vi "MeasureGrowthTrends.vi"(8 "Fixed":T1={"FixedDays"=FALSE, "DaysBack"=7, "FixTrendDays"=FALSE, "DaysBackTrend"=0}, 11 "Data":cluster{"Cases":i32[], "Days":timestamp[]}={"Cases"=[0, 0, 0, 0, 2, 2, 2, 2, 2, 3, 3, 3, 6, 6, 6, 6, 6, 6, 6, 6, 7, 7, 8, 8, 8, 8, 8, 8, 8, 8, 10, 10, 10, 10, 10, 10, 11, 11, 12, 12, 21, 25, 35, 51, 59, 102, 116, 167, 179, 247, 250, 305, 372, 480, 588, 741, 892, 1065, 1289, 1524, 1826, 2253, 2641, 3176, 4035, 4863, 5671, 6352, 7412, 8570, 9939, 11170, 12563, 13886], "Days"=[timestamp(3662524800 s since 1904-01-01), timestamp(3662611200 s since 1904-01-01), timestamp(3662697600 s since 1904-01-01), timestamp(3662784000 s since 1904-01-01), timestamp(3662870400 s since 1904-01-01), timestamp(3662956800 s since 1904-01-01), timestamp(3663043200 s since 1904-01-01), timestamp(3663129600 s since 1904-01-01), timestamp(3663216000 s since 1904-01-01), timestamp(3663302400 s since 1904-01-01), timestamp(3663388800 s since 1904-01-01), timestamp(3663475200 s since 1904-01-01), timestamp(3663561600 s since 1904-01-01), timestamp(3663648000 s since 1904-01-01), timestamp(3663734400 s since 1904-01-01), timestamp(3663820800 s since 1904-01-01), timestamp(3663907200 s since 1904-01-01), timestamp(3663993600 s since 1904-01-01), timestamp(3664080000 s since 1904-01-01), timestamp(3664166400 s since 1904-01-01), timestamp(3664252800 s since 1904-01-01), timestamp(3664339200 s since 1904-01-01), timestamp(3664425600 s since 1904-01-01), timestamp(3664512000 s since 1904-01-01), timestamp(3664598400 s since 1904-01-01), timestamp(3664684800 s since 1904-01-01), timestamp(3664771200 s since 1904-01-01), timestamp(3664857600 s since 1904-01-01), timestamp(3664944000 s since 1904-01-01), timestamp(3665030400 s since 1904-01-01), timestamp(3665116800 s since 1904-01-01), timestamp(3665203200 s since 1904-01-01), timestamp(3665289600 s since 1904-01-01), timestamp(3665376000 s since 1904-01-01), timestamp(3665462400 s since 1904-01-01), timestamp(3665548800 s since 1904-01-01), timestamp(3665635200 s since 1904-01-01), timestamp(3665721600 s since 1904-01-01), timestamp(3665808000 s since 1904-01-01), timestamp(3665894400 s since 1904-01-01), timestamp(3665980800 s since 1904-01-01), timestamp(3666067200 s since 1904-01-01), timestamp(3666153600 s since 1904-01-01), timestamp(3666240000 s since 1904-01-01), timestamp(3666326400 s since 1904-01-01), timestamp(3666412800 s since 1904-01-01), timestamp(3666499200 s since 1904-01-01), timestamp(3666585600 s since 1904-01-01), timestamp(3666672000 s since 1904-01-01), timestamp(3666758400 s since 1904-01-01), timestamp(3666844800 s since 1904-01-01), timestamp(3666931200 s since 1904-01-01), timestamp(3667017600 s since 1904-01-01), timestamp(3667104000 s since 1904-01-01), timestamp(3667190400 s since 1904-01-01), timestamp(3667276800 s since 1904-01-01), timestamp(3667363200 s since 1904-01-01), timestamp(3667449600 s since 1904-01-01), timestamp(3667536000 s since 1904-01-01), timestamp(3667622400 s since 1904-01-01), timestamp(3667708800 s since 1904-01-01), timestamp(3667795200 s since 1904-01-01), timestamp(3667881600 s since 1904-01-01), timestamp(3667968000 s since 1904-01-01), timestamp(3668054400 s since 1904-01-01), timestamp(3668140800 s since 1904-01-01), timestamp(3668227200 s since 1904-01-01), timestamp(3668313600 s since 1904-01-01), timestamp(3668400000 s since 1904-01-01), timestamp(3668486400 s since 1904-01-01), timestamp(3668572800 s since 1904-01-01), timestamp(3668659200 s since 1904-01-01), timestamp(3668745600 s since 1904-01-01), timestamp(3668832000 s since 1904-01-01)]}) -> (0 "Trend":cluster{"Days":timestamp[], dbl[]}[](graph), 1 "Growth":cluster{"Days":timestamp[], dbl[]}[](graph), 3 "Measure":T2={"Trend"=0.0, "TrendBest"=0.0, "TrendWorst"=0.0, "BestDays"=0.0, "WorstDays"=0.0, "Days"=0.0, "Growth"=16.31168636482856, "PlusMinus"=2.4408305776857144, "Cases"=0})   [LabVIEW 2017]
panel:
  out "GrowthError":dbl
  out "Growth":dbl
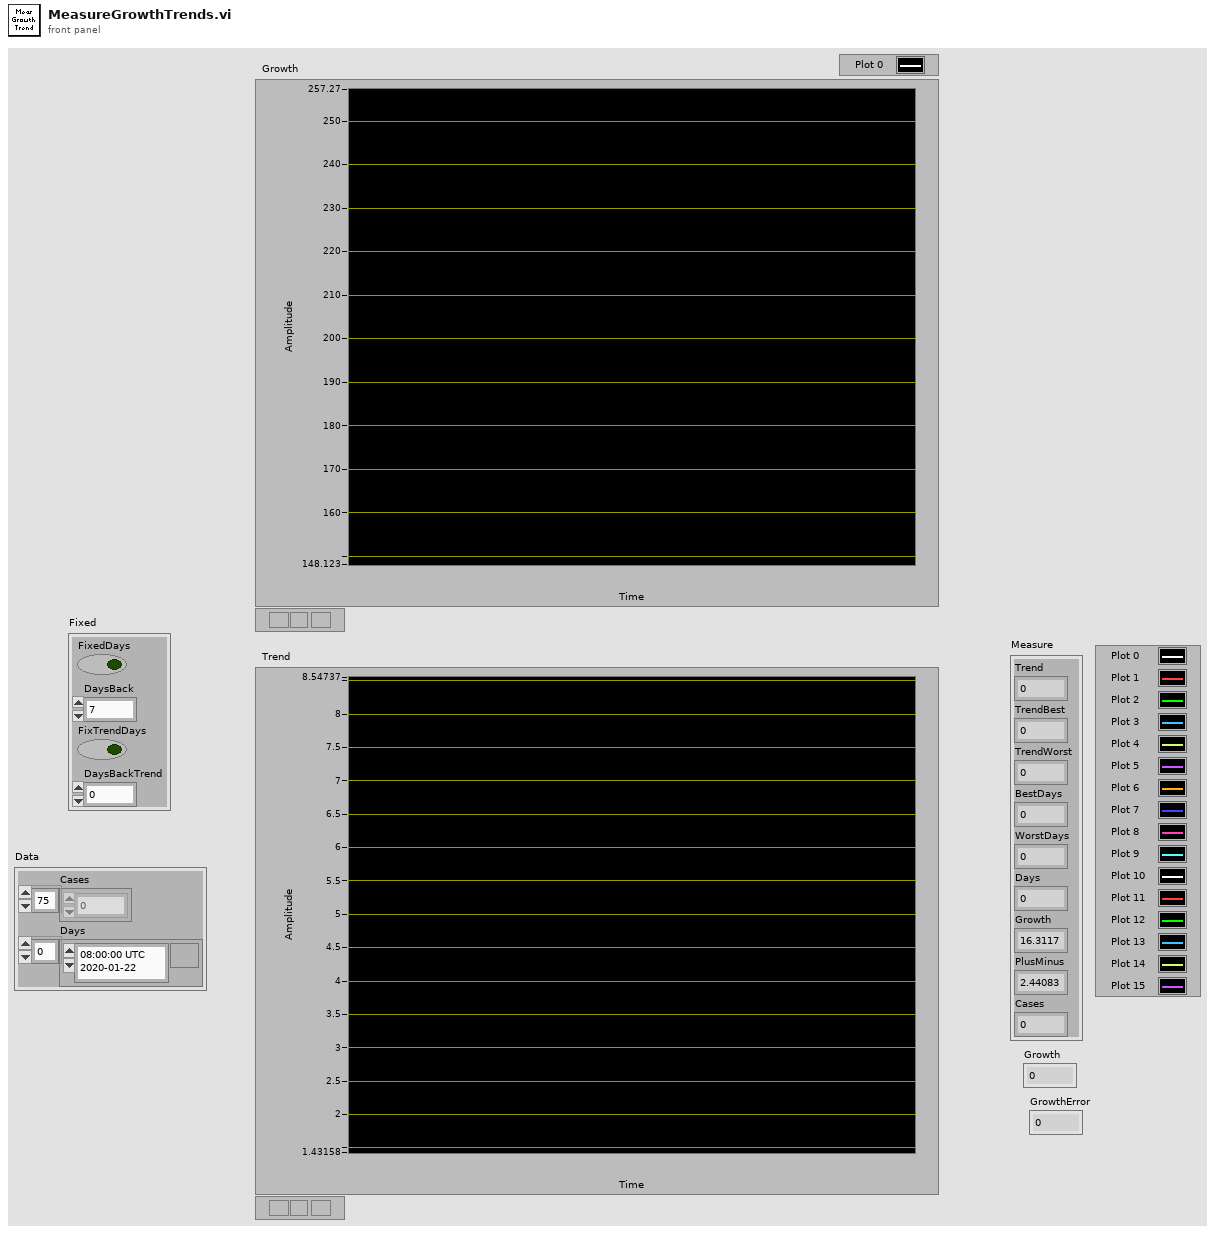
[diagram p1: front panel]
types:
  T1 = cluster{"FixedDays":bool, "DaysBack":i32, "FixTrendDays":bool, "DaysBackTrend":i32}
  T2 = cluster{"Trend":dbl, "TrendBest":dbl, "TrendWorst":dbl, "BestDays":dbl, "WorstDays":dbl, "Days":dbl, "Growth":dbl, "PlusMinus":dbl, "Cases":i32}
  T3 = cluster{"Days":timestamp[], "ConfirmedCases":dbl[]}[]
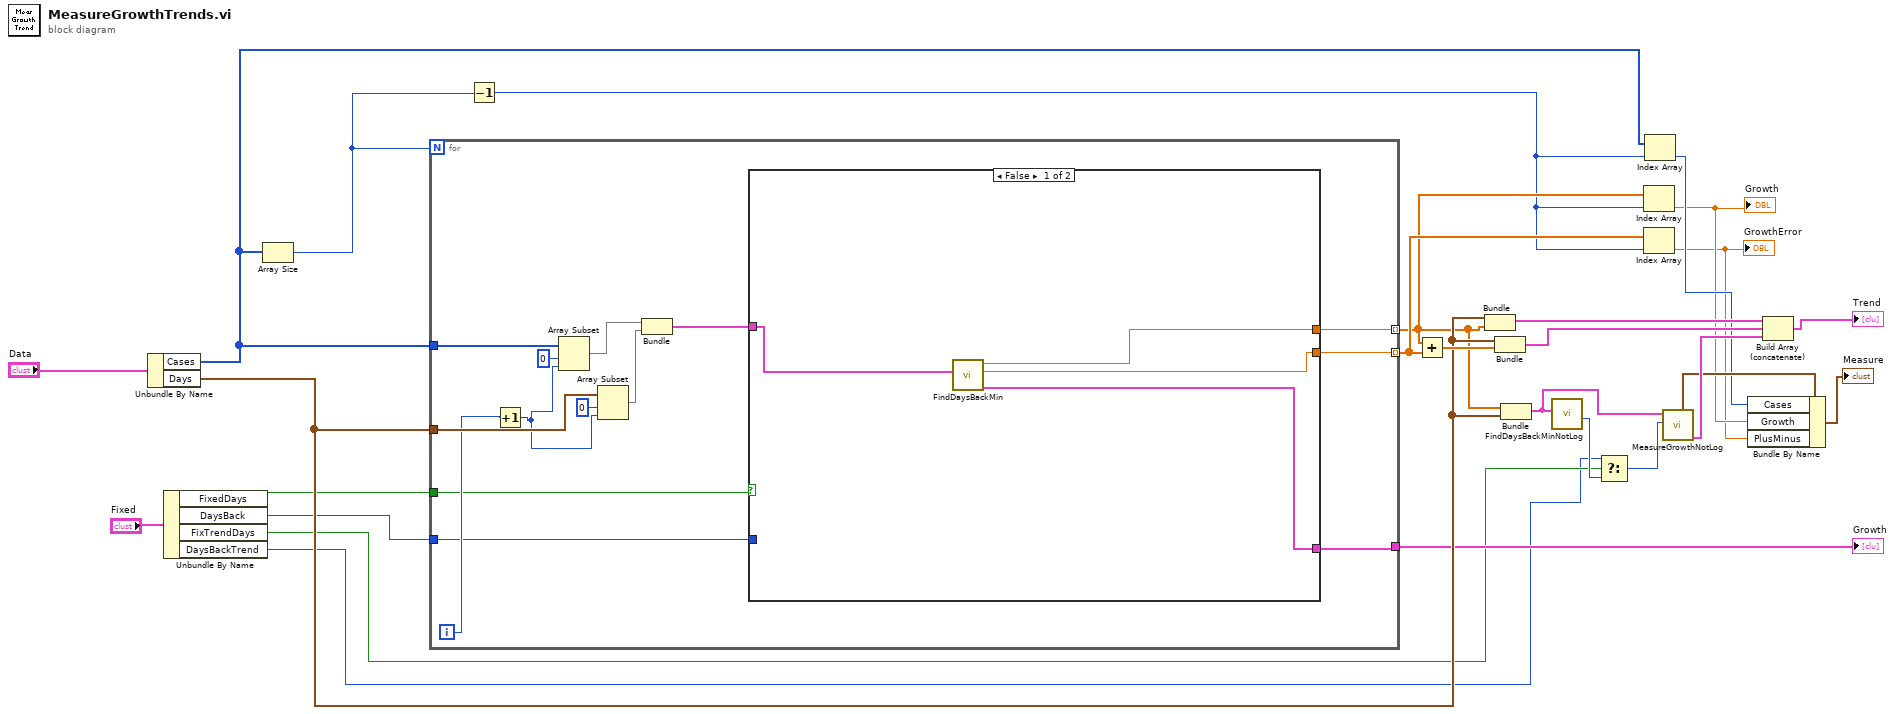
[diagram p0: block diagram]
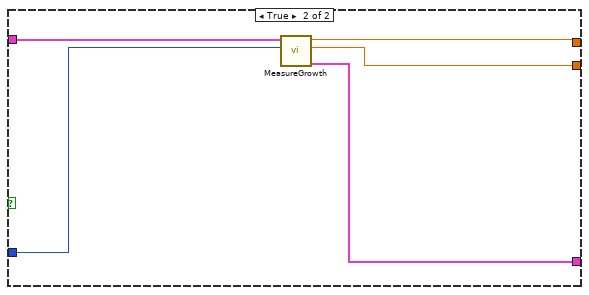
[diagram p2: hidden frame]
diagram:
  n1 = Unbundle By Name("Data") -> ("Cases"=w11:i32[], "Days"=w22:timestamp[])
  n2 = Unbundle By Name("Fixed") -> ("FixedDays"=w4:bool, "DaysBack"=w3:i32, "FixTrendDays"=w2:bool, "DaysBackTrend"=w1:i32)
  n3 = Array Size(array=w11) -> (size(s)=w20:i32)
  n4 = for {
    N: w20 -> [_]
    tunnel: w11 -> [w40]
    tunnel: w22 -> [w37]
    tunnel: [w33] -> w16 mode=indexing
    tunnel: w4 -> [w30]
    tunnel: w3 -> [w29]
    tunnel: [w28] -> w19 mode=indexing
    tunnel: [w27] -> w14
    i -> [w32]
    n5 = Increment(x=w32) -> (x+1=w31:i32)
    n6 = Array Subset(array=w40, index=0, length=w31) -> (w36:i32[])
    n7 = Array Subset(array=w37, index=0, length=w31) -> (w35:timestamp[])
    n8 = Bundle(w36, w35) -> (w34:cluster{i32[], timestamp[]})  [unwired: 1 in]
    n9 = case shown="False" w30 {
      tunnel: w34 -> [w44 w49]
      tunnel: [w43 w47] -> w33
      tunnel: w29 -> [_ w48]
      tunnel: [w42 w46] -> w28
      tunnel: [w41 w45] -> w27
      frame False {
        n10 = call "FindDaysBackMin.vi"("Cluster"=w44) -> ("Plot"=w41:T3, "Error"=w42:dbl, "Growth"=w43:dbl)  [unwired: 7 in, 1 out]
      }
      frame True {
        n11 = call "MeasureGrowth.vi"("DaysBack"=w48, "Data"=w49) -> ("Plot"=w45:T3, "PlusMinus"=w46:dbl, "Growth"=w47:dbl)  [unwired: 4 in, 3 out]
      }
    }
  }
  "Growth" <- w14
  n12 = Decrement(x=w20) -> (x-1=w10:i32)
  n13 = Add(x=w16, y=w19) -> (x+y=w26:dbl[])
  n14 = Bundle("Days"=w22, w16) -> (w24:cluster{"Days":timestamp[], dbl[]})  [unwired: 1 in]
  n15 = Bundle("Days"=w22, w26) -> (w25:cluster{"Days":timestamp[], dbl[]})  [unwired: 1 in]
  n16 = Bundle(w16, "Days"=w22) -> (w21:cluster{dbl[], "Days":timestamp[]})  [unwired: 1 in]
  n17 = call "FindDaysBackMinNotLog.vi"("Cluster"=w21) -> ("Index"=w18:i32)  [unwired: 8 in, 2 out]
  n18 = Select(t=w1, s=w2, f=w18) -> (s? t:f=w17:i32)
  n19 = Index Array(array=w16, index=w10) -> (element=w7:dbl)
  "Growth" <- w7
  n20 = Index Array(array=w19, index=w10) -> (element=w6:dbl)
  "GrowthError" <- w6
  n21 = Index Array(array=w11, index=w10) -> (element=w9:i32)
  n22 = call "MeasureGrowthNotLog.vi"("DaysBack"=w17, "Data"=w21) -> ("Plot"=w15:T3, "Measure"=w12:T2)  [unwired: 3 in, 5 out]
  n23 = Bundle By Name(cluster=w12, "Cases"=w9, "Growth"=w7, "PlusMinus"=w6) -> (→"Measure":T2)
  n24 = Build Array (concatenate)(w24, w25, w15) -> (→"Trend":T3)
